vi "Run (hybrid).vi"(8 "error in (no error)":errorcluster, 9 "Array of States LUT":variant[](array[variant]), 10 "States LUT (name -> boolean state)":variant, 11 "TriggerAction in":refnum<class "TriggerAction Q.lvclass">) -> (0 "error out":errorcluster, 3 "TriggerAction out":refnum<class "TriggerAction Q.lvclass">)   [LabVIEW 2016, in "TriggerAction Q.lvclass"]
uses:
  <userlib>/Common Components/TriggerAction Q/TriggerAction Q/TriggerAction Q.lvclass
  <userlib>/Common Components/TriggerAction Q/TriggerAction Q/TriggerAction Q.lvclass/TriggerAction Q.ctl
  <userlib>/Common Components/Function Messages/Action Dispatch Msg/Action Dispatch Msg.lvclass/Action Dispatch Msg.ctl
  <vilib>/ActorFramework/Message Enqueuer/Message Enqueuer.lvclass/Message Enqueuer.ctl
  <vilib>/ActorFramework/Message Enqueuer/Enqueue.vi
  <userlib>/Common Components/Function Messages/Action Dispatch Msg/Action Dispatch Msg.lvclass
  C:/Program Files (x86)/National Instruments/LabVIEW 2016/vi.lib/ActorFramework/Message/Message.lvclass
  <vilib>/ActorFramework/Message Priority Queue/Priority Enqueue.vi
panel:
  # "System level states"
  # "States of each motion"
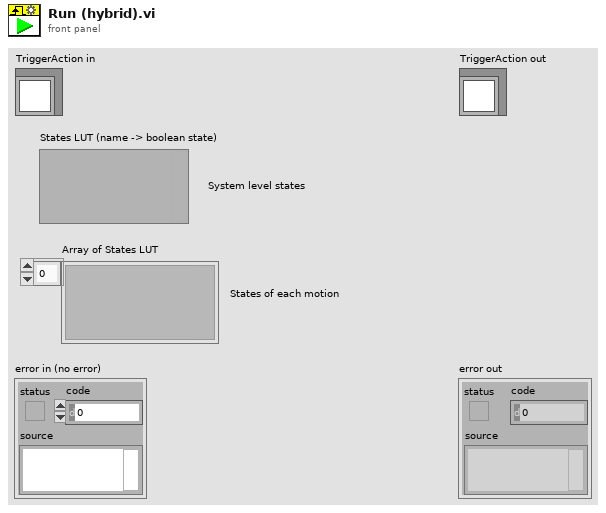
[diagram p1: front panel]
types:
  T1 = typedef "TriggerAction.lvclass/Element Data.ctl" = cluster{"Triggers":cluster{"Triggers for Array AND":string[]}[], "Actions":cluster{"Action Name":string, "Action Data":string}[]}
  T2 = cluster{"Action Name":string, "Action Data":string}[]
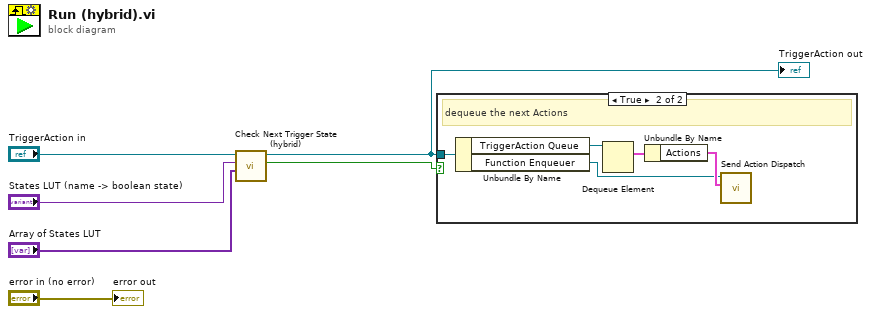
[diagram p0: block diagram]
diagram:
  n1 = call <userlib>:"Check Next Trigger State (hybrid).vi"("Array of States LUT"="Array of States LUT", "States LUT (name -> boolean state)"="States LUT (name -> boolean state)", "TriggerAction in"="TriggerAction in") -> ("Trigger State"=w4:bool, "TriggerAction out"=w3:refnum<class "TriggerAction Q.lvclass">)  [unwired: 6 in, 1 out]
  "TriggerAction out" <- w3
  n2 = case shown="True" w4 {
    tunnel: w3 -> [_ w11]
    frame False {
    }
    frame True {
      # "dequeue the next Actions"
      n3 = Unbundle By Name(w11) -> ("TriggerAction Queue"=w10:refnum<queue>, "Function Enqueuer"=w7:refnum<class "Message Enqueuer.lvclass">)
      n4 = Dequeue Element(queue=w10) -> (element=w9:T1)  [unwired: 2 in, 3 out]
      n5 = Unbundle By Name(w9) -> ("Actions"=w8:T2)
      n6 = call <userlib>:"Send Action Dispatch.vi"("Actions"=w8, "Message Enqueuer"=w7) -> ()  [unwired: 8 in, 2 out]
    }
  }
  "error out" <- "error in (no error)"
